vi "Initialize UI core.vi"(8 "error in (no error)":errorcluster, 11 "Dialog in":refnum<class "Dialog.lvclass">) -> (0 "error out":errorcluster, 1 "Autoshow?":bool, 2 "Panel Updater":refnum<class "Panel Updater.lvclass">, 3 "Dialog out":refnum<class "Dialog.lvclass">)   [LabVIEW 2017, in "MGI-Panel Manager.lvlib" / "Dialog.lvclass"]
doc: "Opens the dialog UI and sets it to modal.\n\n----\nPlease see the following web address for additional documentation and tutorial information:\nhttp://www.mooregoodideas.com/mgi-panel-manager/\n\nAuthor: Derek Trepanier\n\nCopyright (c) 2018, Moore Good Ideas, Inc.\n\nAll rights reserved.\n\nRedistribution and use in source and binary forms, with or without modification, are permitted provided that the following conditions are met:\n\n * Redistributions of source code must retain the above copyright notice, this list of conditions and the following disclaimer.\n * Redistributions in binary form must reproduce the above copyright notice, this list of conditions and the following disclaimer in the documentation and/or other materials provided with the distribution.\n * Neither the name of Moore Good Ideas, Inc. nor the names of its contributors may be used to endorse or promote products derived from this software without specific prior written permission.\n\nTHIS SOFTWARE IS PROVIDED BY THE COPYRIGHT HOLDERS AND CONTRIBUTORS \"AS IS\" AND ANY EXPRESS OR IMPLIED WARRANTIES, INCLUDING, BUT NOT LIMITED TO, THE IMPLIED WARRANTIES OF MERCHANTABILITY AND FITNESS FOR A PARTICULAR PURPOSE ARE DISCLAIMED. IN NO EVENT SHALL THE COPYRIGHT OWNER OR CONTRIBUTORS BE LIABLE FOR ANY DIRECT, INDIRECT, INCIDENTAL, SPECIAL, EXEMPLARY, OR CONSEQUENTIAL DAMAGES (INCLUDING, BUT NOT LIMITED TO, PROCUREMENT OF SUBSTITUTE GOODS OR SERVICES; LOSS OF USE, DATA, OR PROFITS; OR BUSINESS INTERRUPTION) HOWEVER CAUSED AND ON ANY THEORY OF LIABILITY, WHETHER IN CONTRACT, STRICT LIABILITY, OR TORT (INCLUDING NEGLIGENCE OR OTHERWISE) ARISING IN ANY WAY OUT OF THE USE OF THIS SOFTWARE, EVEN IF ADVISED OF THE POSSIBILITY OF SUCH DAMAGE."
uses:
  Dialog.lvclass
  D:/software/LabView_PanelManager/panel-manager/Source/Panel/Panel.lvclass
  Panel Updater/Panel Updater.lvclass
  Panel.lvclass/Panel.ctl
  Dialog.lvclass/Dialog.ctl
  Window.lvclass
  Panel.lvclass
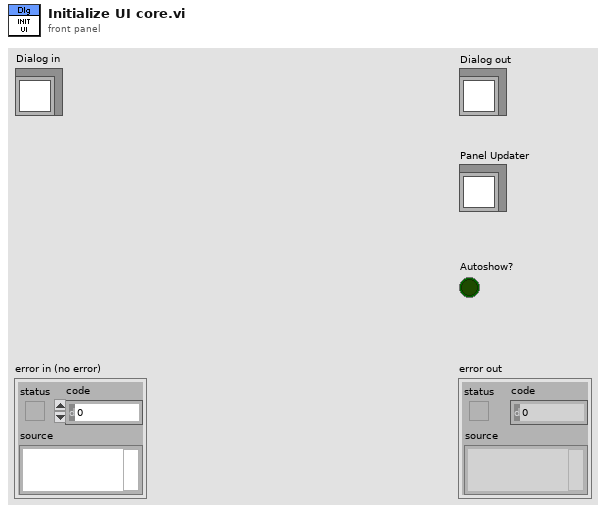
[diagram p1: front panel]
types:
  T1 = typedef "MGI-Panel Manager.lvlib/Dialog.lvclass/Behavior.ctl" = enum32{"Floating", "Floating/Auto-Hide", "Modal"}
  T2 = enum32{"Invalid", "Default", "Floating", "Floating/Auto-Hide", "Modal"}
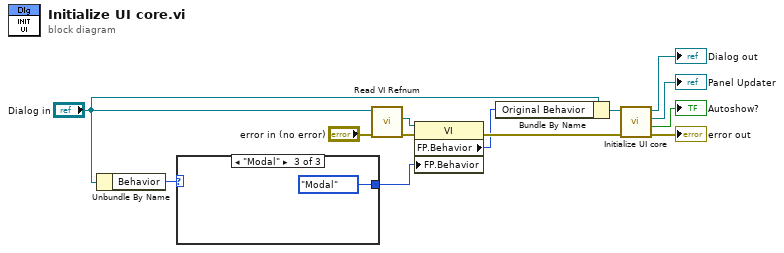
[diagram p0: block diagram]
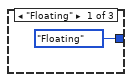
[diagram p2: hidden frame]
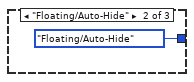
[diagram p3: hidden frame]
diagram:
  n1 = Unbundle By Name("Dialog in") -> ("Behavior"=w4:T1)
  n2 = case shown="\"Modal\"" w4 {
    tunnel: [T2."Floating" ("Front Panel Window:Behavior") T2."Floating/Auto-Hide" ("Front Panel Window:Behavior") T2."Modal" ("Front Panel Window:Behavior")] -> w3
    frame "Floating" {
    }
    frame "Floating/Auto-Hide" {
    }
    frame "Modal" {
    }
  }
  n3 = call "Read VI Refnum.vi"("error in (no error)"="error in (no error)", "Panel in"="Dialog in") -> ("error out"=w10:errorcluster, "VI Refnum"=w11:refnum<vi>)  [unwired: 8 in]
  n4 = property class="VI"(reference=w11, error in=w10, "FP.Behavior"=w3) -> (error out=w9:errorcluster, "FP.Behavior"=w6:T2)  [unwired: 1 out]
  n5 = Bundle By Name(cluster="Dialog in", "Original Behavior"=w6) -> (w7:refnum<class "Dialog.lvclass">)
  n6 = call-parent "Initialize UI core.vi"("error in (no error)"=w9, "Window in"=w7) -> ("error out"=→"error out":errorcluster, "Autoshow?"=→"Autoshow?":bool, "Panel Updater"=→"Panel Updater":refnum<class "Panel Updater.lvclass">, "Window out"=→"Dialog out":refnum<class "Dialog.lvclass">)  [unwired: 6 in]
